vi "HVSConvertStringToData.vi"(8 "error in (no error)":errorcluster, 11 "String":string) -> (0 "error out":errorcluster, 2 "Valid Data":bool, 3 "value":dbl[](array[numeric]))   [LabVIEW 2013]
panel:
  # "Report Date Time, Barometric Pressure (mmHg), Ambient Temperature (°C)\n, Wind speed (m/s), Wind direction (°), Sigma Theta (standard deviation for wind direction), \nRainfall (bucket tips), Flow-rate (m3/h), Corrected accumulated sample volume (standard m3), \nUncorrected accumulated sample volume (m3)"
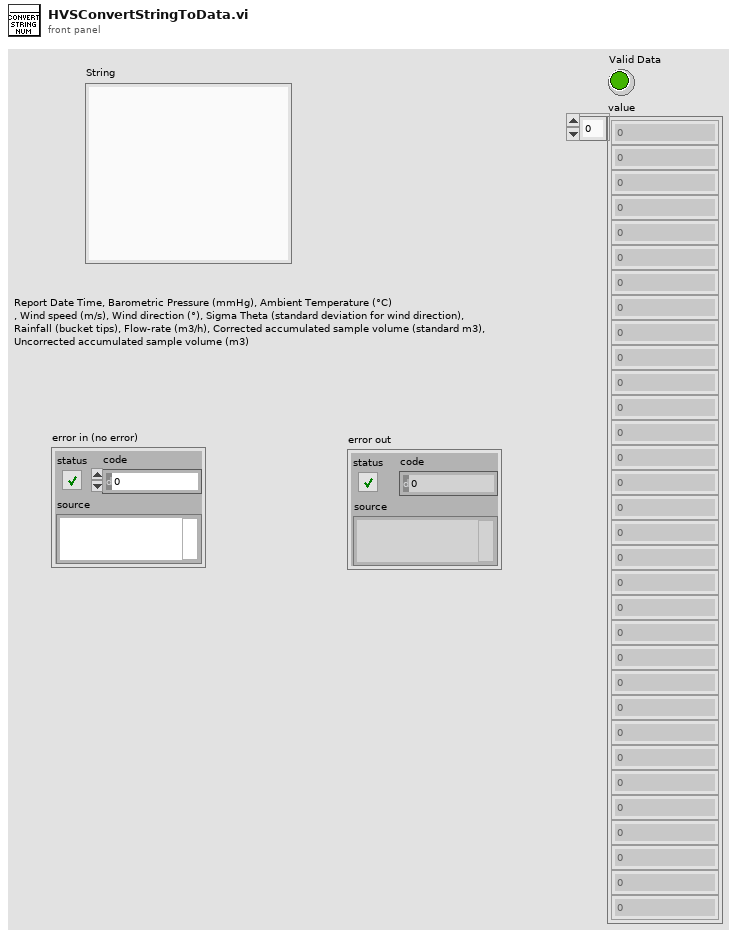
[diagram p1: front panel]
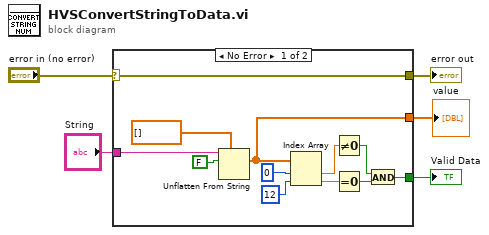
[diagram p0: block diagram]
diagram:
  n1 = case shown="No Error" "error in (no error)" {
    selector: "error in (no error)" -> [w8 w18]
    tunnel: "String" -> [w9 _]
    tunnel: [w8 w18] -> w3
    tunnel: [w7 _] -> w2
    tunnel: [w6 _] -> w1
    frame No Error {
      n2 = Unflatten From String(type=sgl[] [], binary string=w9, data includes array or string size? (T)=FALSE) -> (value=w6:sgl[])  [unwired: 2 in, 2 out]
      n3 = Index Array(array=w6, index #1=0 ("index"), index #2=12 ("index")) -> (element #1=w14:sgl, element #2=w11:sgl)
      n4 = Not Equal To 0?(x=w14) -> (x != 0?=w13:bool)
      n5 = Equal To 0?(x=w11) -> (x = 0?=w10:bool)
      n6 = And(x=w13, y=w10) -> (x .and. y?=w7:bool)
    }
    frame Error {
    }
  }
  "error out" <- w3
  "Valid Data" <- w2
  "value" <- w1
